vi "ccd_triggeredmovieacquire_bkup.vi"() -> ()   [LabVIEW 2009]
panel:
  out "output path":path
  out "Y 3":dbl
  out "X 3":dbl
  out "Y 2":dbl
  out "X 2":dbl
  out "Image 2":T1(plugin-control)
  out "Image":T1(plugin-control)
  out "cameraName":dbl
  out "imageType":dbl
  out "trigger_number":dbl
  out "framenumber":dbl
  out "Y":dbl
  out "X":dbl
  in  "Trigger action":u32(ring)=1 items=["Disabled", "Trigger start of acquisition", "Trigger start of each buffer list", "Trigger each buffer", "Trigger each line (linescan)", "Trigger end of acquisition"]
  in  "Trigger Type":u32(ring) items=["External", "RTSI", "ISO In"]
  in  "Data frames / trigger":dbl=10.0
  in  "Video Frames / Data frame":dbl=15.0
  in  "GO":bool
  in  "stop":bool
  in  "Manual (up) or automatic (down)":bool
  in  "Or, read path automatically from:":path=path "\\\\Foghorn.bio.brandeis.edu\\remote"
  in  "Manual save directory":string
  in  "Manual save path":path
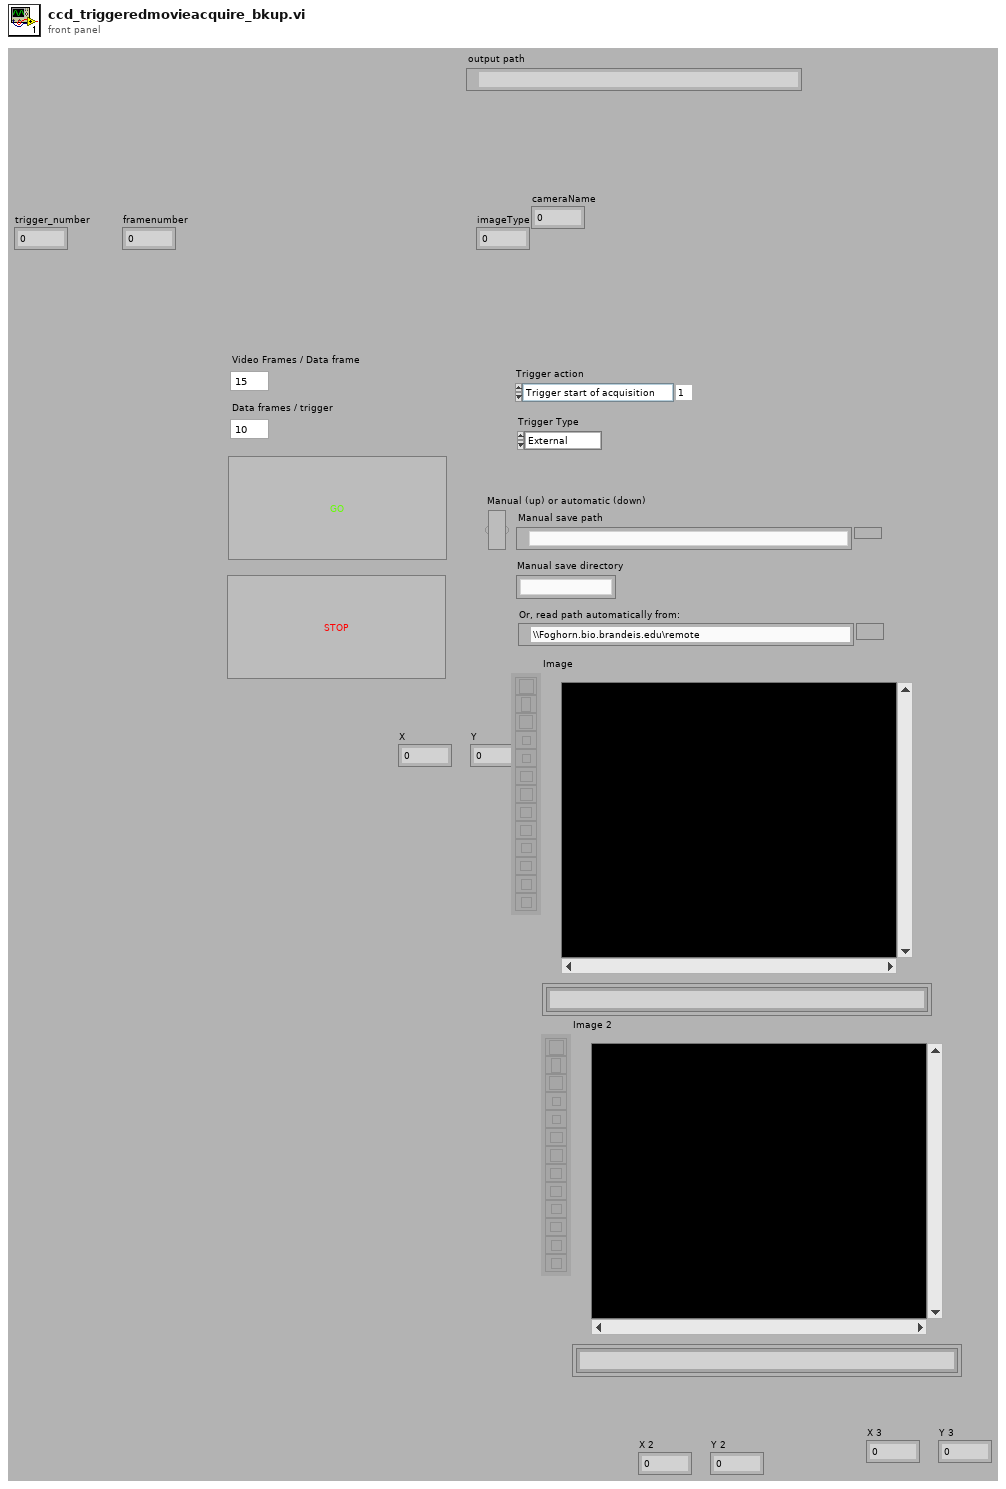
[diagram p1: front panel]
types:
  T1 = typedef "IMAQ Image.ctl" = refnum<image>
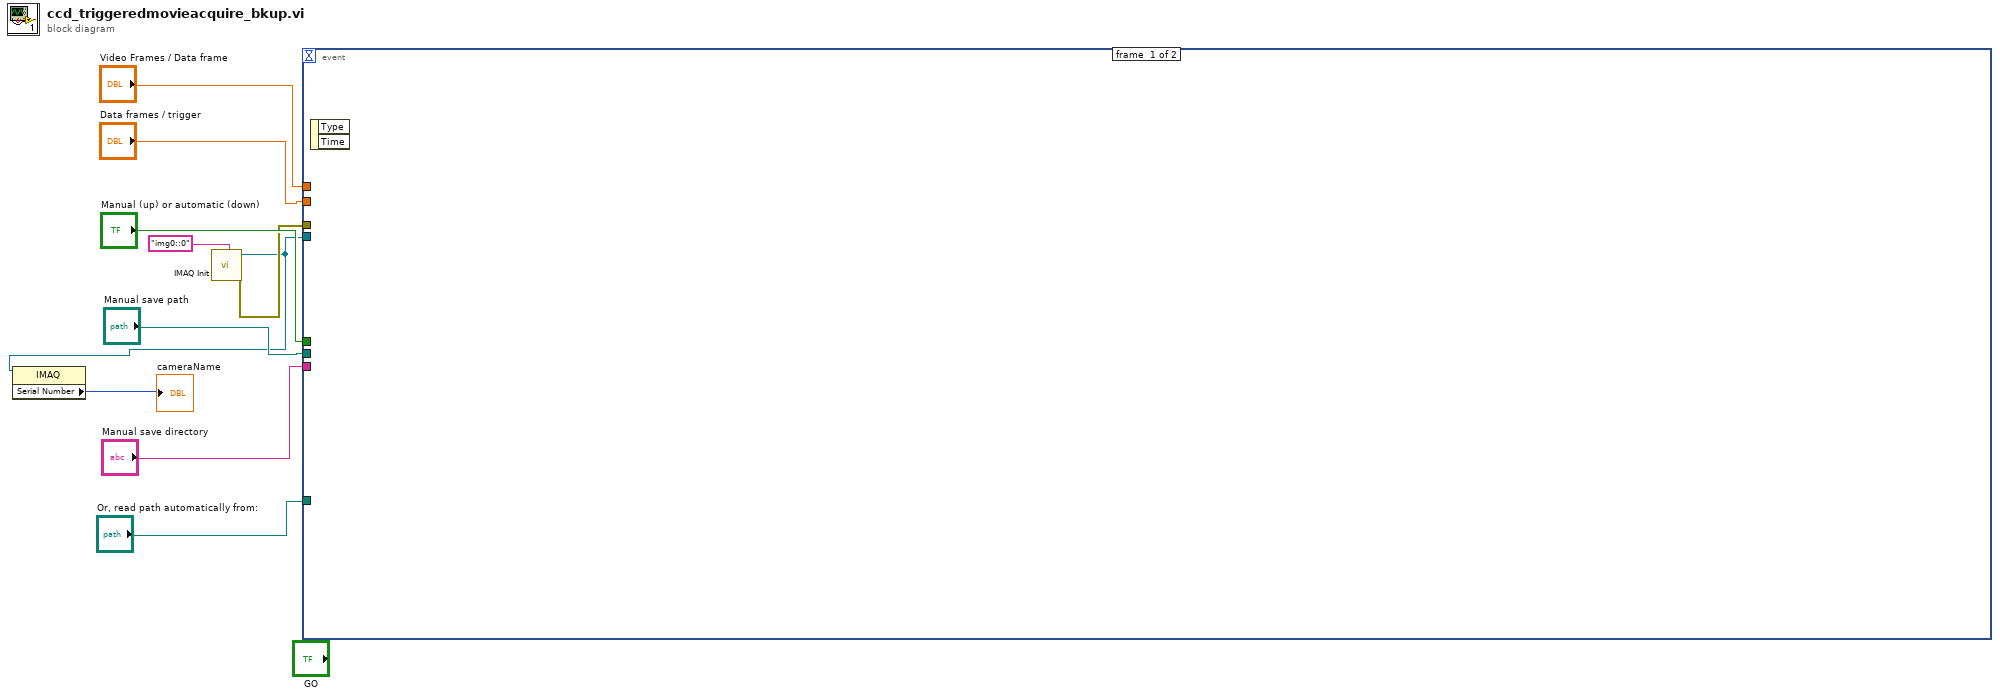
[diagram p0: block diagram]
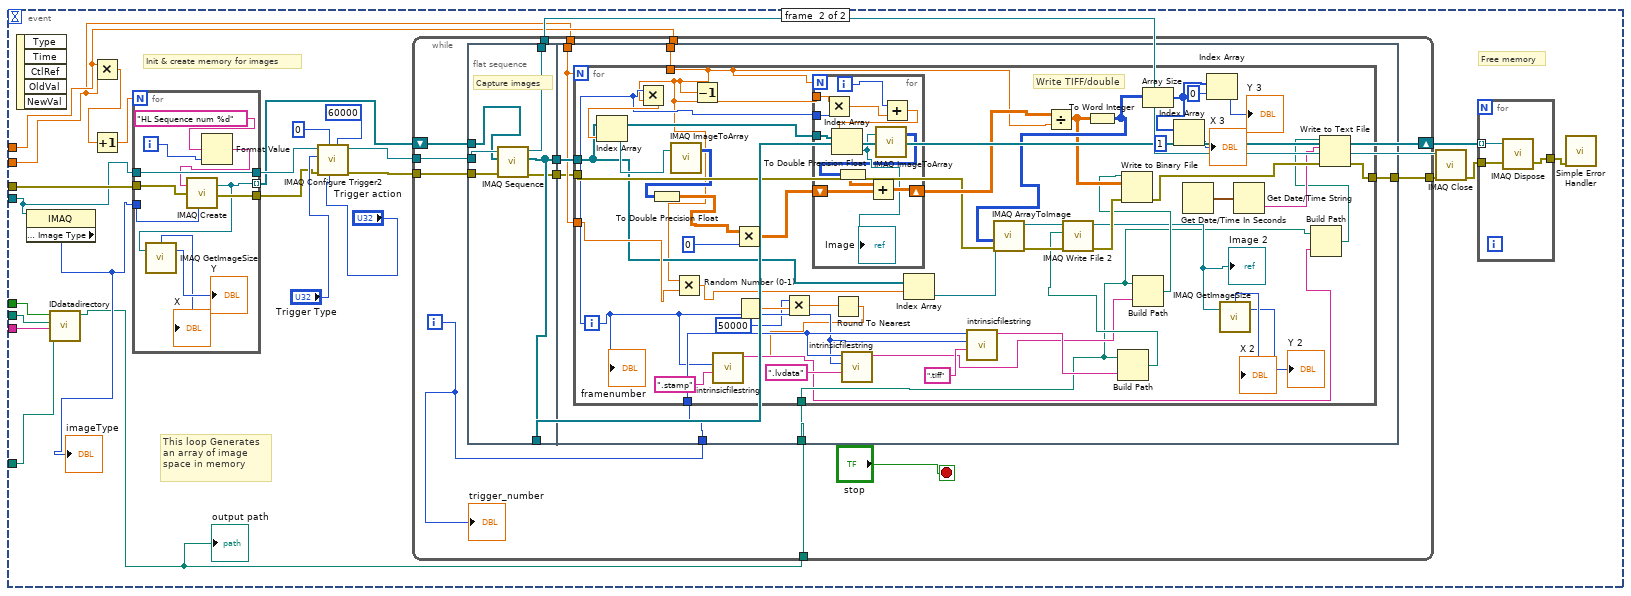
[diagram p2: hidden frame]
diagram:
  n1 = call <vilib>:"IMAQ Init.vi"("Interface Name"="img0::0") -> ("error out"=w4:errorcluster, "IMAQ Session Out"=w2:refnum<k11>)  [unwired: 9 in]
  n2 = property class="IMAQ"(reference=w2) -> ("Serial Number"=→"cameraName":u32)  [unwired: 1 in, 2 out]
  n3 = event shown="[1] \"GO\": Value Change" {
    selector: _ -> [_ _]
    dyn-events: _ -> [_ _]
    timeout: _ -> [_ _]
    tunnel: "Video Frames / Data frame" -> [_ w23]
    tunnel: "Data frames / trigger" -> [_ w22]
    tunnel: "Or, read path automatically from:" -> [_ w27]
    tunnel: "Manual save directory" -> [_ w26]
    tunnel: "Manual save path" -> [_ w25]
    tunnel: "Manual (up) or automatic (down)" -> [_ w24]
    tunnel: w4 -> [_ w15]
    tunnel: w2 -> [_ w14]
    event #0 {
      n4 = event-data() -> ()  [unwired: 1 in, 2 out]
    }
    event #1 {
      # "Free memory"
      # "This loop Generates an array of image space in memory"
      # "Init & create memory for images"
      n5 = event-data() -> ()  [unwired: 1 in, 5 out]
      n6 = property class="IMAQ"(reference=w14) -> ("Image Parameters : Image Type"=w13:u32)  [unwired: 1 in, 2 out]
      "imageType" <- w13
      n7 = call "IDdatadirectory.vi"("Read path automatically from:"=w27, "Directory"=w26, "Save path"=w25, "Manual or automatic"=w24) -> ("Outputpath"=w11:path)  [unwired: 7 in]
      "output path" <- w11
      n8 = Multiply(x=w23, y=w22) -> (x*y=w21:dbl)
      n9 = Increment(x=w21) -> (x+1=w20:dbl)
      n10 = for {
        N: w20 -> [_]
        tunnel: [w132] -> w32
        tunnel: [w128] -> w19 mode=indexing
        tunnel: w15 -> [w131]
        tunnel: w14 -> [w130]
        tunnel: [w130] -> w33
        tunnel: w13 -> [w129]
        i -> [w124]
        n11 = Format Value(format string="HL Sequence num %d", value (0)=w124) -> (output string=w123:string)  [unwired: 1 in]
        n12 = call "IMAQ Create"("Image Name"=w123, "Image Type"=w129, "error in (no error)"=w131) -> ("New Image"=w128:T1, "error out"=w132:errorcluster)  [unwired: 2 in]
        n13 = call "IMAQ GetImageSize"("Image"=w128) -> ("Y Resolution"=→"Y":i32, "X Resolution"=→"X":i32)  [unwired: 3 in, 1 out]
      }
      n14 = call <vilib>:"IMAQ Configure Trigger2.vi"("Frame timeout (ms)"=u32 60000, "Trigger action"="Trigger action", "Trigger Polarity"=0, "error in (no error)"=w32, "Trigger Type"="Trigger Type", "IMAQ Session In"=w33) -> ("error out"=w30:errorcluster, "IMAQ Session Out"=w31:refnum<k11>)  [unwired: 4 in]
      n15 = while {
        tunnel: w31 -> [w52]
        tunnel: w30 -> [w51]
        shift-right: [w43] -> w18
        shift-left: w19 -> [w45]
        tunnel: [w49] -> w28
        tunnel: w11 -> [w48]
        tunnel: w23 -> [w47]
        tunnel: w22 -> [w46]
        tunnel: [w41] -> w17
        i -> [w40]
        stop <- "stop" stop-if-true
        n16 = flat-sequence {
          tunnel: w52 -> [w56]
          tunnel: w51 -> [w58]
          tunnel: [w54] -> w50
          tunnel: [w57] -> w49
          tunnel: w45 -> [w55]
          tunnel: [w54] -> w43
          tunnel: [w53] -> w42
          tunnel: w50 -> [w65]
          tunnel: w48 -> [w64]
          tunnel: w40 -> [w59]
          tunnel: w47 -> [w63]
          tunnel: w46 -> [w62]
          tunnel: w42 -> [w61]
          tunnel: [w60] -> w41
          frame #0 {
            # "Capture images"
            n17 = call <vilib>:"IMAQ Sequence.vi"("error in (no error)"=w58, "Images In"=w55, "IMAQ Session In"=w56) -> ("error out"=w53:errorcluster, "Images Out"=w54:T1[], "IMAQ Session Out"=w57:refnum<k11>)  [unwired: 6 in]
          }
          frame #1 {
            n18 = for {
              N: w62 -> [_]
              tunnel: w65 -> [w70]
              tunnel: w64 -> [w81]
              tunnel: w59 -> [w83]
              tunnel: w63 -> [w66]
              tunnel: w62 -> [w109]
              tunnel: w61 -> [w106]
              tunnel: [w79] -> w60
              i -> [w82]
              # "Write TIFF/double"
              n19 = Multiply(x=w82, y=w66) -> (x*y=w110:dbl)
              n20 = Index Array(array=w70, index=w110) -> (element=w111:T1)
              n21 = call "IMAQ ImageToArray"("Image"=w111) -> ("Image Pixels (I16)"=w96:i16[][])  [unwired: 3 in, 4 out]
              n22 = To Double Precision Float(number=w96) -> (double precision float=w69:dbl[][])
              n23 = Multiply(x=w66, y=w109) -> (x*y=w107:dbl)
              n24 = Decrement(x=w66) -> ()  [unwired: 1 out]
              n25 = Multiply(x=w69, y=0) -> (x*y=w68:dbl[][])
              n26 = Random Number (0-1)() -> (number: 0 to 1=w74:dbl)
              n27 = Multiply(x=50000, y=w74) -> (x*y=w72:dbl)
              n28 = for {
                N: w66 -> [_]
                tunnel: w70 -> [w122]
                shift-right: [w119] -> w108
                shift-left: w68 -> [w120]
                tunnel: w66 -> [w118]
                tunnel: w82 -> [w117]
                i -> [w113]
                n29 = Multiply(x=w118, y=w117) -> (x*y=w116:dbl)
                n30 = Add(x=w113, y=w116) -> (x+y=w112:dbl)
                n31 = Index Array(array=w122, index=w112) -> (element=w115:T1)
                "Image" <- w115
                n32 = call "IMAQ ImageToArray"("Image"=w115) -> ("Image Pixels (I16)"=w114:i16[][])  [unwired: 3 in, 4 out]
                n33 = To Double Precision Float(number=w114) -> (double precision float=w121:dbl[][])
                n34 = Add(x=w121, y=w120) -> (x+y=w119:dbl[][])
              }
              n35 = Round To Nearest(number=w72) -> (nearest integer value=w71:dbl)
              n36 = call "intrinsicfilestring.vi"("Postfix"=".stamp", "Frame number"=w82, "Trigger number"=w71) -> ("Filestring"=w80:string)  [unwired: 8 in]
              n37 = call "intrinsicfilestring.vi"("Postfix"=".lvdata", "Frame number"=w82, "Trigger number"=w83) -> ("Filestring"=w87:string)  [unwired: 8 in]
              n38 = Index Array(array=w70, index=w107) -> (element=w92:T1)
              n39 = call "intrinsicfilestring.vi"("Postfix"=".tiff", "Frame number"=w82, "Trigger number"=w83) -> ("Filestring"=w94:string)  [unwired: 8 in]
              n40 = Divide(x=w108, y=w66) -> (x/y=w88:dbl[][])
              n41 = To Word Integer(number=w88) -> (16bit integer=w95:i16[][])
              n42 = call "IMAQ ArrayToImage"("error in (no error)"=w106, "Image Pixels (I16)"=w95, "Image"=w92) -> ("error out"=w105:errorcluster, "Image Out"=w104:T1)  [unwired: 7 in]
              n43 = Build Path(base path=w81, name or relative path=w94) -> (appended path=w91:path)
              n44 = call-poly "IMAQ Write File 2"("error in (no error)"=w105, "File Path"=w91, "Image"=w104) -> ("error out"=w89:errorcluster, "Image Out (duplicate)"=w85:T1)  [unwired: 7 in]
              "Image 2" <- w85
              n45 = Build Path(base path=w81, name or relative path=w87) -> (appended path=w86:path)
              n46 = Write to Binary File(file (use dialog)=w86, data=w88, error in=w89) -> (error out=w78:errorcluster)  [unwired: 3 in, 2 out]
              n47 = Array Size(array=w95) -> (size(s)=w100:i32[])
              n48 = Index Array(array=w100, index=1) -> (element=→"X 3":i32)
              n49 = Get Date/Time In Seconds() -> (seconds since 1Jan1904=w75:timestamp)
              n50 = Index Array(array=w100, index=0) -> (element=→"Y 3":i32)
              n51 = call "IMAQ GetImageSize"("Image"=w85) -> ("Y Resolution"=→"Y 2":i32, "X Resolution"=→"X 2":i32)  [unwired: 3 in, 1 out]
              n52 = Get Date/Time String(seconds (now)=w75) -> (time string=w77:string)  [unwired: 2 in, 1 out]
              n53 = Build Path(base path=w81, name or relative path=w80) -> (appended path=w76:path)
              n54 = Write to Text File(file (use dialog)=w76, text=w77, error in=w78) -> (error out=w79:errorcluster)  [unwired: 1 in, 2 out]
              "framenumber" <- w82
            }
          }
        }
        "trigger_number" <- w40
      }
      n55 = call <vilib>:"IMAQ Close.vi"("error in (no error)"=w17, "IMAQ Session In"=w28) -> ("error out"=w16:errorcluster)  [unwired: 9 in]
      n56 = for {
        tunnel: w18 -> [w39] mode=indexing
        tunnel: w16 -> [w38]
        tunnel: [w37] -> w29
        n57 = call "IMAQ Dispose"("Image"=w39, "error in (no error)"=w38) -> ("error out"=w37:errorcluster)  [unwired: 4 in]
      }
      n58 = call <vilib>:"Simple Error Handler.vi"("error in (no error)"=w29) -> ()  [unwired: 4 in, 5 out]
    }
  }
